vi "Init.vi"(9 "Request":refnum<class "Request.lvclass">, 10 "Client":refnum<class "Client.lvclass">, 11 "OAuth2 in (New)":refnum<class "OAuth2.lvclass">) -> (3 "OAuth2":refnum<class "OAuth2.lvclass">)   [LabVIEW 2020, in "OAuth2.lvlib" / "OAuth2.lvclass"]
doc: "Initializes the mechanism to requets user authorization via OAuth2 Authorization Code Flow. The Client input determines the application client credentials that have been created with the desired authorization platform and the Request input defines the URLs and how the auth flow is performed."
uses:
  OAuth2.lvclass
  Client/Client.lvclass
  Request/Request.lvclass
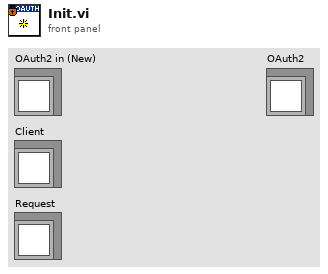
[diagram p1: front panel]
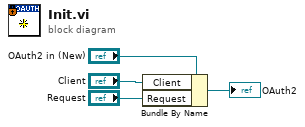
[diagram p0: block diagram]
diagram:
  n1 = Bundle By Name(cluster="OAuth2 in (New)", "Client"="Client", "Request"="Request") -> (→"OAuth2":refnum<class "OAuth2.lvclass">)
